vi "SelectTubel.vi"(8 "error in (no error)":errorcluster, 10 "Unique Object Identifier":string, 11 "DataHandler in":refnum<class "DataHandlerMYiTOPS.lvclass">) -> (0 "error out":errorcluster, 2 "Array":string[][](array[string]), 3 "DataHandler out":refnum<class "DataHandlerMYiTOPS.lvclass">)   [LabVIEW 2015, in "DataHandlerMYiTOPS.lvclass"]
uses:
  DataHandlerMYiTOPS.lvclass
  <vilib>/drjdpowell/SQLite Library/SQL Statement/SQL Statement.lvclass
  <vilib>/drjdpowell/SQLite Library/SQL Connection/Connection.lvclass
panel:
  # "1 - 'Activity (on / off)', \n2 - 'Prioritization', \n3 - 'El. Power Limitation',  \n4 - 'Th. Power Limitation',\n5 - 'Release Time'"
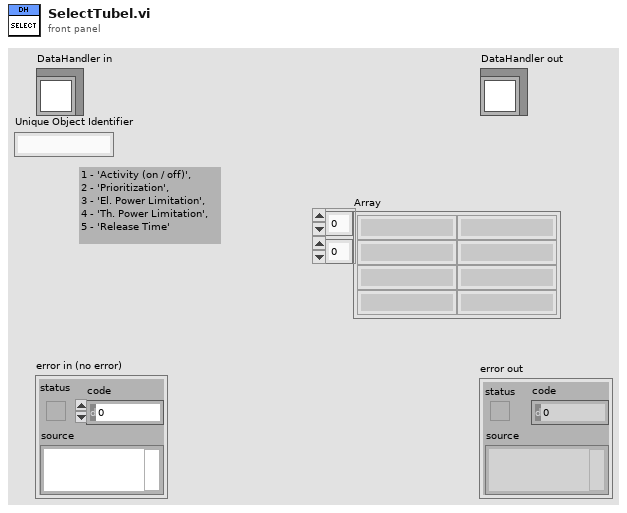
[diagram p1: front panel]
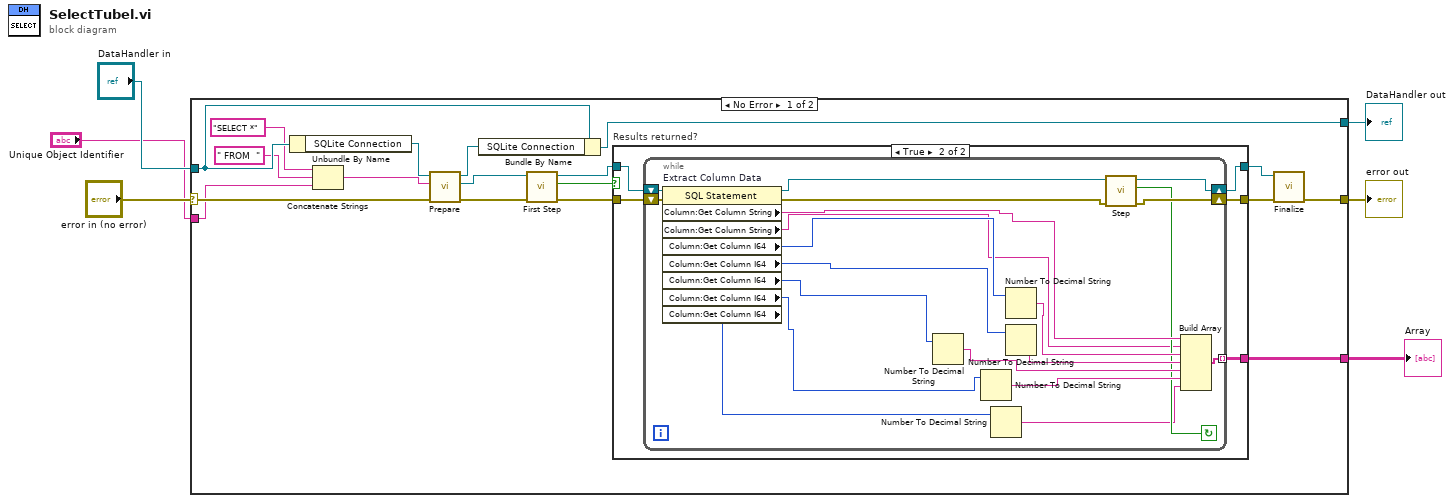
[diagram p0: block diagram]
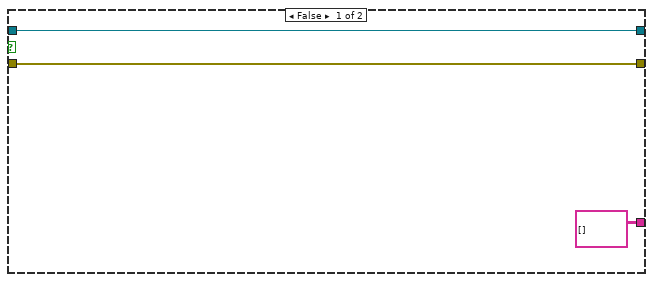
[diagram p2: hidden frame]
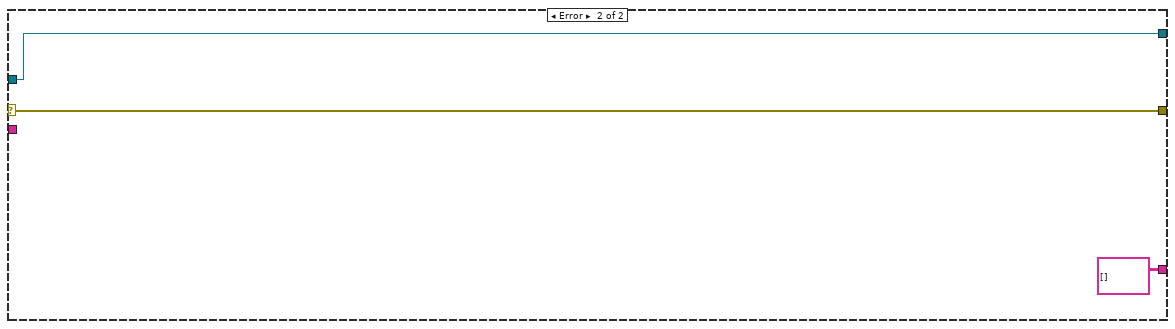
[diagram p3: hidden frame]
diagram:
  n1 = case shown="No Error" "error in (no error)" {
    selector: "error in (no error)" -> [w13 w55]
    tunnel: [w12 w55] -> w5
    tunnel: [w15 w54] -> w3
    tunnel: "DataHandler in" -> [w16 w54]
    tunnel: "Unique Object Identifier" -> [w10 _]
    tunnel: [w7 string[][] []] -> w1
    frame No Error {
      n2 = Unbundle By Name(w16) -> ("SQLite Connection"=w17:refnum<class "Connection.lvclass">)
      n3 = Concatenate Strings("SELECT *" ("string"), " FROM  " ("string"), w10) -> (w9:string)
      n4 = call <vilib>:"Prepare.vi"("error in (no error)"=w13, "SQL"=w9, "SQLite Connection in"=w17) -> ("error out"=w18:errorcluster, "SQL Statement out"=w19:refnum<class "SQL Statement.lvclass">, "SQLite Connection out"=w14:refnum<class "Connection.lvclass">)  [unwired: 4 in, 2 out]
      n5 = Bundle By Name(cluster=w16, "SQLite Connection"=w14) -> (w15:refnum<class "DataHandlerMYiTOPS.lvclass">)
      n6 = call <vilib>:"First Step.vi"("error in (no error)"=w18, "SQL Statement in"=w19) -> ("error out"=w21:errorcluster, "Row returned"=w20:bool, "SQL Statement out"=w22:refnum<class "SQL Statement.lvclass">)  [unwired: 7 in]
      n7 = case "Results returned?" shown="True" w20 {
        tunnel: [w27 w29] -> w23
        tunnel: [w26 w30] -> w24
        tunnel: w22 -> [w27 w32]
        tunnel: w21 -> [w26 w31]
        tunnel: [string[][] [] w28] -> w7
        frame False {
        }
        frame True {
          n8 = while {
            tunnel: [w50] -> w28 mode=indexing
            shift-right: [w37] -> w29
            shift-left: w32 -> [w52]
            shift-right: [w38] -> w30
            shift-left: w31 -> [w51]
            stop <- w36 continue-if-true
            n9 = property on="Extract Column Data" class="SQL Statement"(reference=w52, error in=w51) -> (reference out=w40:refnum<class "SQL Statement.lvclass">, error out=w39:errorcluster, "Column:Get Column String"=w49:string, "Column:Get Column String"=w35:string, "Column:Get Column I64"=w48:i64, "Column:Get Column I64"=w46:i64, "Column:Get Column I64"=w42:i64, "Column:Get Column I64"=w41:i64, "Column:Get Column I64"=w34:i64)
            n10 = Number To Decimal String(number=w42) -> (decimal integer string=w44:string)  [unwired: 1 in]
            n11 = Number To Decimal String(number=w41) -> (decimal integer string=w43:string)  [unwired: 1 in]
            n12 = Number To Decimal String(number=w34) -> (decimal integer string=w33:string)  [unwired: 1 in]
            n13 = Number To Decimal String(number=w48) -> (decimal integer string=w47:string)  [unwired: 1 in]
            n14 = Number To Decimal String(number=w46) -> (decimal integer string=w45:string)  [unwired: 1 in]
            n15 = call <vilib>:"Step.vi"("error in (no error)"=w39, "SQL Statement in"=w40) -> ("error out"=w38:errorcluster, "Row returned"=w36:bool, "SQL Statement out"=w37:refnum<class "SQL Statement.lvclass">)  [unwired: 7 in]
            n16 = Build Array(w49, w35, w47, w45, w44, w43, w33) -> (w50:string[])
          }
        }
      }
      n17 = call <vilib>:"Finalize.vi"("error in (no error)"=w24, "SQL Statement in"=w23) -> ("error out"=w12:errorcluster)  [unwired: 9 in]
    }
    frame Error {
    }
  }
  "error out" <- w5
  "DataHandler out" <- w3
  "Array" <- w1
